vi "CCM-Read DODI Connection Tables.vi"(0 "Path In":path, 11 "error in (no error)":errorcluster) -> (4 "Path Out":path, 8 "Tables":cluster{"Table":T1[]}[](array[cluster]), 15 "error out":errorcluster)   [LabVIEW 2020]
uses:
  Type Defs/CM-Connection.ctl
  Type Defs/CM-IO Type.ctl
  Utility VIs/File IO VIs/Configuration File Wrapper VIs/Config-Read Key (string).vi
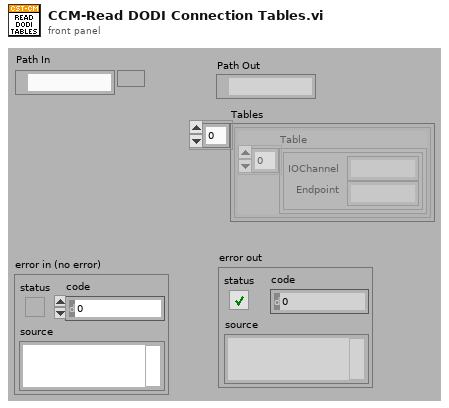
[diagram p1: front panel]
types:
  T1 = typedef "CM-Connection.ctl" = cluster{"IOChannel":string, "Endpoint":string}
  T2 = typedef "CM-IO Type.ctl" = enum16{"Analog Outputs", "Analog Inputs", "Digital Outputs", "Digital Inputs"}
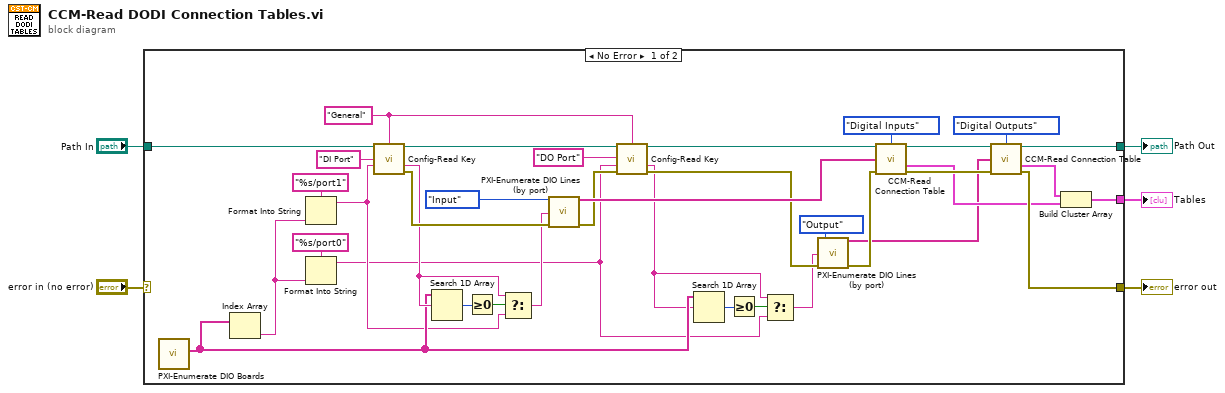
[diagram p0: block diagram]
diagram:
  n1 = case shown="No Error" "error in (no error)" {
    selector: "error in (no error)" -> [_ w44]
    tunnel: "Path In" -> [w28 w43]
    tunnel: [w41 w44] -> w3
    tunnel: [w42 w43] -> w2
    tunnel: [w40 _] -> w1
    frame No Error {
      w30 = "General" ("section")
      n2 = call "PXI-Enumerate DIO Boards.vi"() -> ("Devices"=w11:tag[])  [unwired: 10 in, 1 out]
      n3 = Index Array(array=w11) -> (element=w9:tag)  [unwired: 1 in]
      n4 = Format Into String(format string="%s/port1" ("default"), w9) -> (resulting string=w7:string)  [unwired: 2 in, 1 out]
      n5 = Format Into String(format string="%s/port0" ("default"), w9) -> (resulting string=w6:string)  [unwired: 2 in, 1 out]
      n6 = call-poly "Config-Read Key.vi"("configuration file path"=w28, "section"=w30, "key"="DI Port", "default"=w7) -> ("file path"=w33:path, "value"=w15:string, "error out"=w25:errorcluster)  [unwired: 8 in, 1 out]
      n7 = Search 1D Array(1D array=w11, element=w15) -> (index of element=w17:i32)  [unwired: 1 in]
      n8 = Greater Or Equal To 0?(x=w17) -> (x >= 0?=w16:bool)
      n9 = Select(t=w15, s=w16, f=w7) -> (s? t:f=w14:string)
      n10 = call "PXI-Enumerate DIO Lines (by port).vi"("Direction"=enum16{"Input", "Output"}."Input", "Port"=w14, "error in (no error)"=w25) -> ("Lines"=w26:string[], "error out"=w24:errorcluster)  [unwired: 10 in, 1 out]
      n11 = call-poly "Config-Read Key.vi"("configuration file path"=w33, "section"=w30, "key"="DO Port", "default"=w6, "error in (no error)"=w24) -> ("file path"=w29:path, "value"=w10:string, "error out"=w23:errorcluster)  [unwired: 7 in, 1 out]
      n12 = Search 1D Array(1D array=w11, element=w10) -> (index of element=w13:i32)  [unwired: 1 in]
      n13 = Greater Or Equal To 0?(x=w13) -> (x >= 0?=w12:bool)
      n14 = Select(t=w10, s=w12, f=w6) -> (s? t:f=w8:string)
      n15 = call "PXI-Enumerate DIO Lines (by port).vi"("Direction"=enum16{"Input", "Output"}."Output", "Port"=w8, "error in (no error)"=w23) -> ("Lines"=w20:string[], "error out"=w21:errorcluster)  [unwired: 10 in, 1 out]
      n16 = call "CCM-Read Connection Table.vi"("Path In"=w29, "Type"=CM-IO_Type."Digital Inputs", "IOChannels"=w26, "error in (no error)"=w21) -> ("Path Out"=w37:path, "Table"=w34:T1[], "error out"=w36:errorcluster)  [unwired: 8 in, 1 out]
      n17 = call "CCM-Read Connection Table.vi"("Path In"=w37, "Type"=CM-IO_Type."Digital Outputs", "IOChannels"=w20, "error in (no error)"=w36) -> ("Path Out"=w42:path, "Table"=w35:T1[], "error out"=w41:errorcluster)  [unwired: 8 in, 1 out]
      n18 = Build Cluster Array(w35, w34) -> (w40:cluster{"Table":T1[]}[])
    }
    frame Error {
    }
  }
  "error out" <- w3
  "Path Out" <- w2
  "Tables" <- w1
